vi "SbigWaitIdle.vi"(8 "error in (no error)":errorcluster, 11 "Sbig Name":string) -> (0 "error out":errorcluster, 3 "Sbig Name Out":string)   [LabVIEW 2009]
uses:
  Controls/SbigStatus.ctl
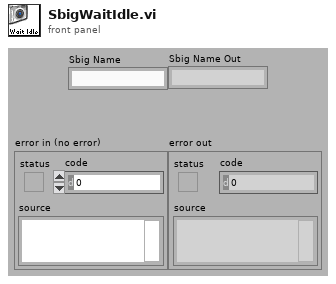
[diagram p1: front panel]
types:
  T1 = typedef "SbigStatus.ctl" = cluster{"Managed ?":bool, "State":enum16{"IDLE", "EXPOSING", "READING"}, "Image":i32[][], "Temperature Info":cluster{"Temperature Regulation":bool, "T Setpoint":dbl, "T CCD":dbl, "T Ambient":dbl, "Cooling %":dbl}}
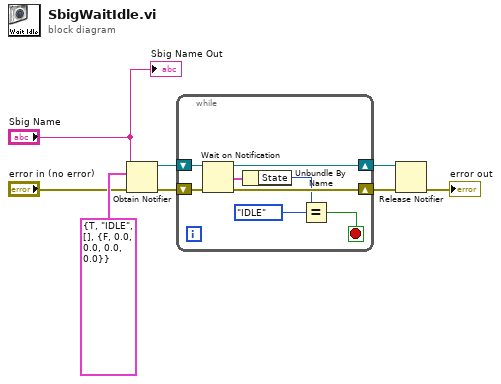
[diagram p0: block diagram]
diagram:
  n1 = Obtain Notifier(name (unnamed)="Sbig Name", notification data type=T1 {"Managed ?"=TRUE, "State"=enum."IDLE", "Image"=[], "Temperature Info"={"Temperature Regulation"=FALSE, "T Setpoint"=0.0, "T CCD"=0.0, "T Ambient"=0.0, "Cooling %"=0.0}} ("Axis Status"), error in (no error)="error in (no error)") -> (notifier out=w4:refnum<notifier>, error out=w5:errorcluster)  [unwired: 1 in, 1 out]
  n2 = while {
    shift-right: [w15] -> w3
    shift-left: w5 -> [w16]
    shift-right: [w9] -> w1
    shift-left: w4 -> [w14]
    stop <- w10 stop-if-true
    n3 = Wait on Notification(notifier=w14, error in (no error)=w16) -> (notifier out=w9:refnum<notifier>, notification=w13:T1, error out=w15:errorcluster)  [unwired: 3 out]
    n4 = Unbundle By Name(w13) -> ("State"=w11:enum16{"IDLE", "EXPOSING", "READING"})
    n5 = Equal?(x=w11, y=enum16{"IDLE", "EXPOSING", "READING"}."IDLE" ("State")) -> (x = y?=w10:bool)
  }
  n6 = Release Notifier(notifier=w1, error in (no error)=w3) -> (error out=→"error out":errorcluster)  [unwired: 3 out]
  "Sbig Name Out" <- "Sbig Name"
